vi "Return_DesiredAngle.vi"(0 "X-Position":dbl, 2 "Y-Position":dbl, 3 "Current Angle":dbl, 9 "Mining Complete":bool) -> (11 "Commence Dumping":bool, 14 "RFM":i32, 15 "RMM":i32, 16 "RRM":i32, 17 "LFM":i32, 18 "LMM":i32, 19 "LRM":i32)   [LabVIEW 2014]
panel:
  out "Desired Angle":dbl
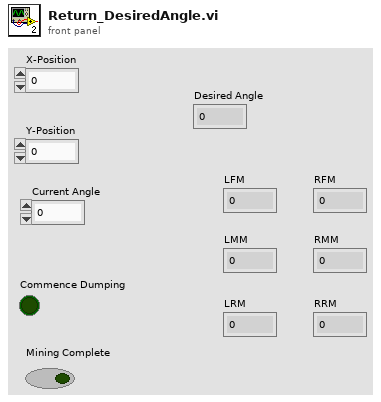
[diagram p1: front panel]
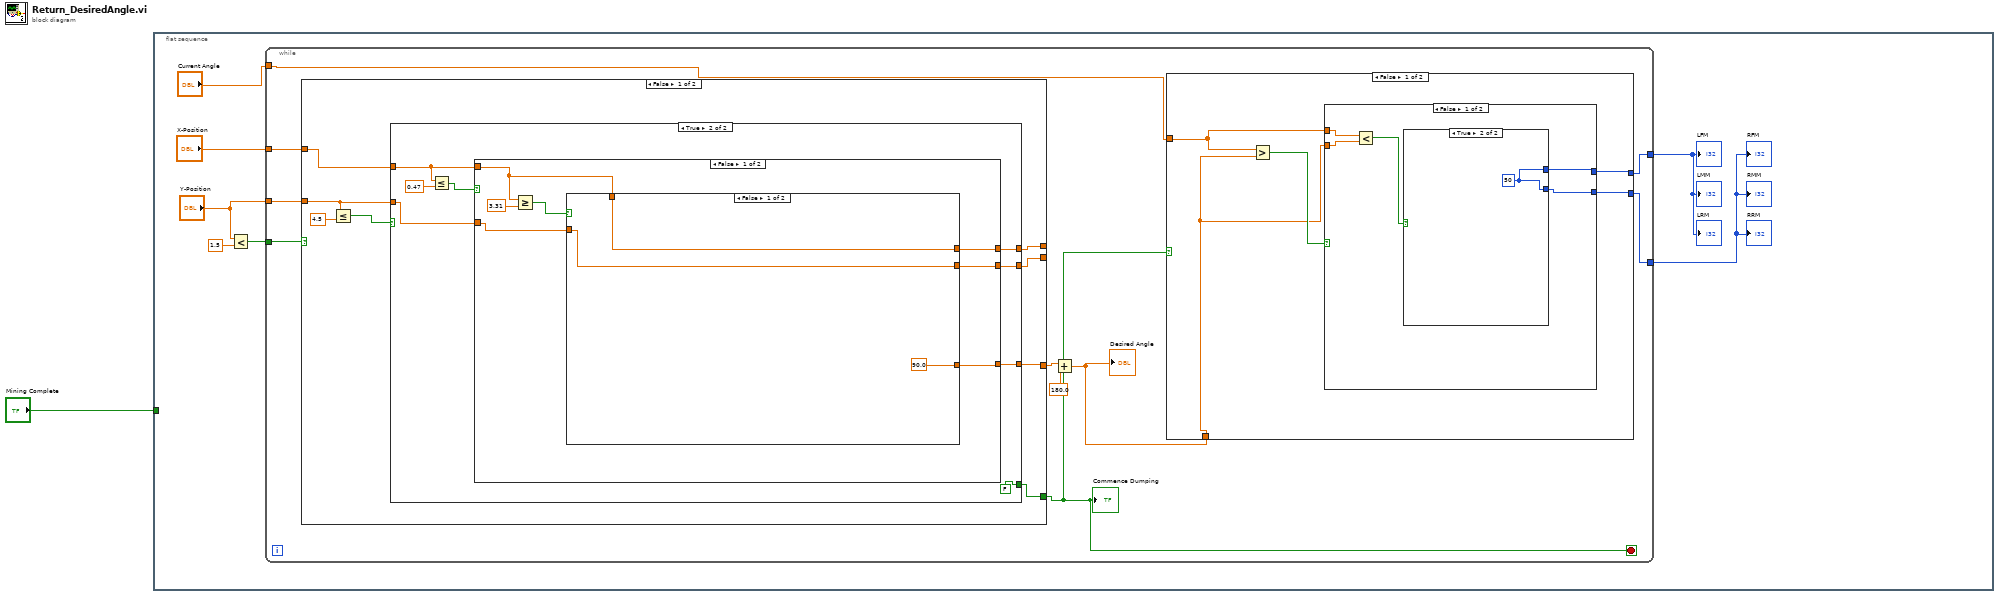
[diagram p0: block diagram]
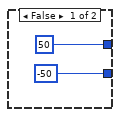
[diagram p2: hidden frame]
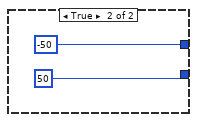
[diagram p3: hidden frame]
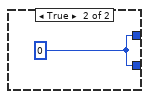
[diagram p4: hidden frame]
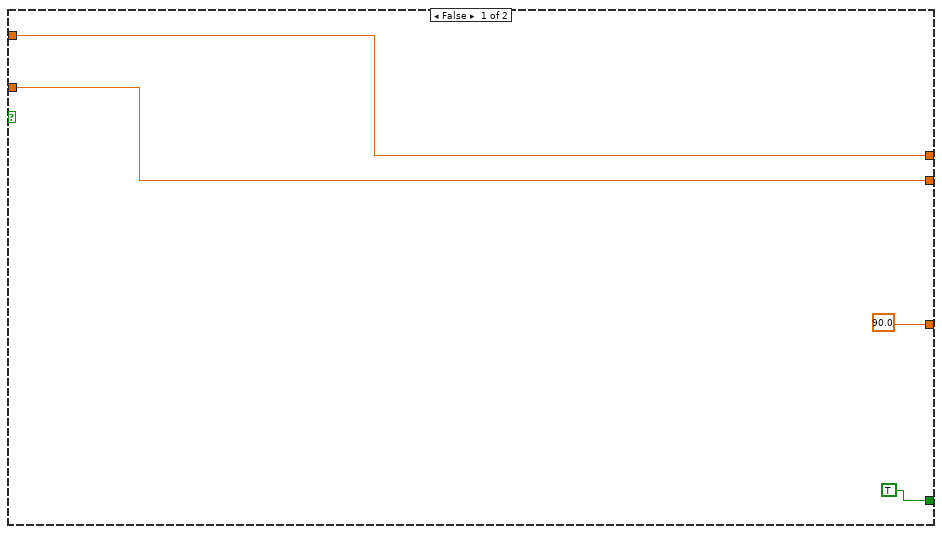
[diagram p5: hidden frame]
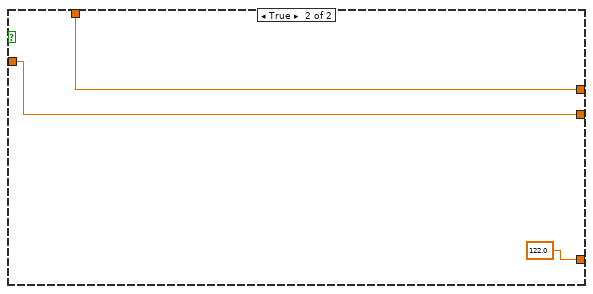
[diagram p6: hidden frame]
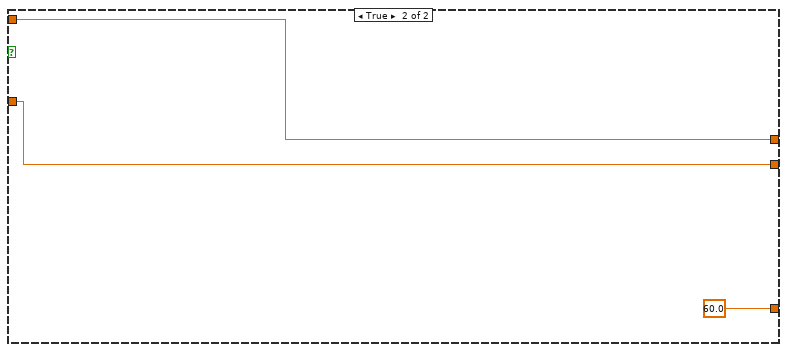
[diagram p7: hidden frame]
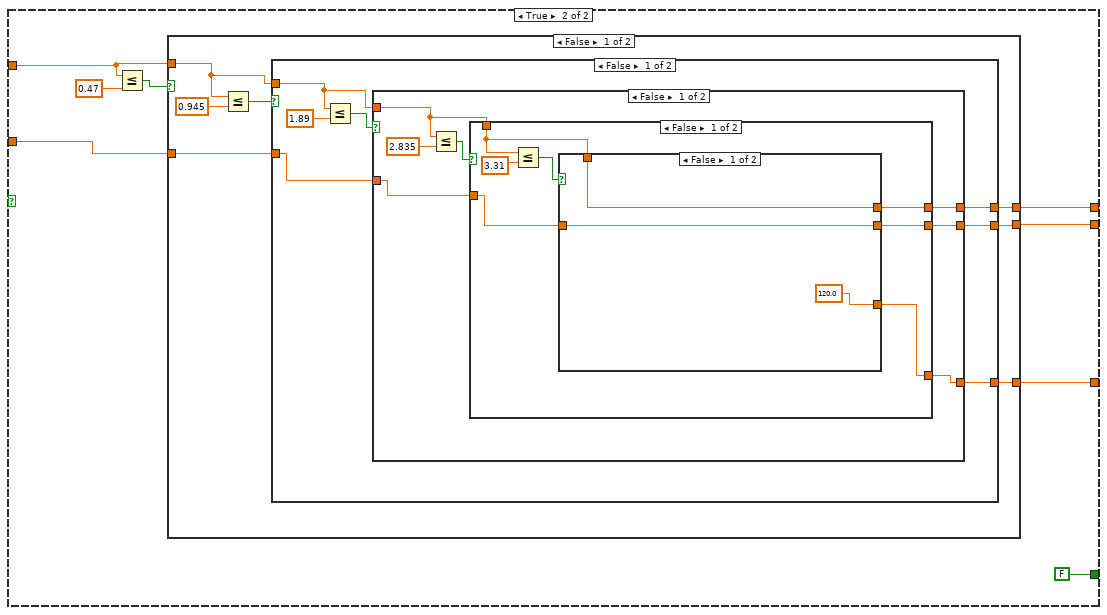
[diagram p8: hidden frame]
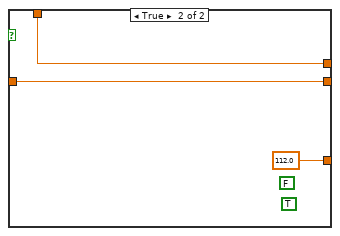
[diagram p9: hidden frame]
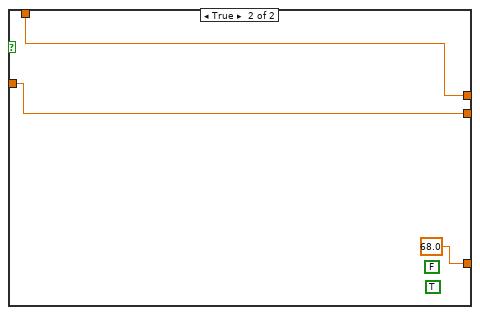
[diagram p10: hidden frame]
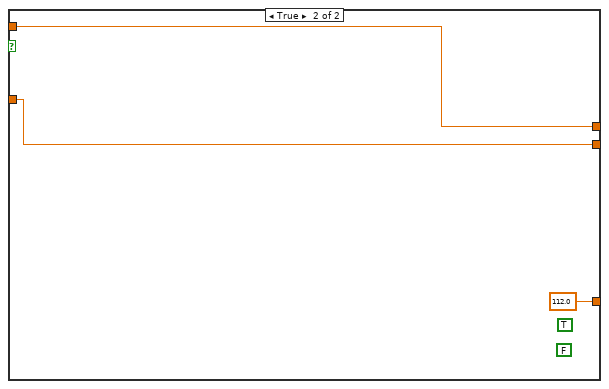
[diagram p11: hidden frame]
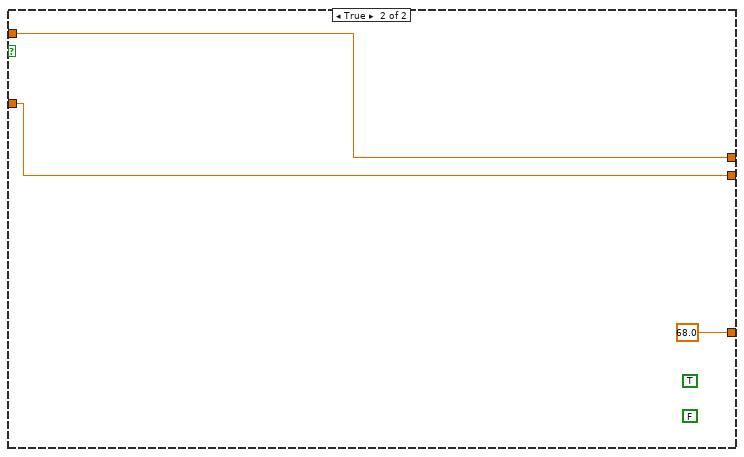
[diagram p12: hidden frame]
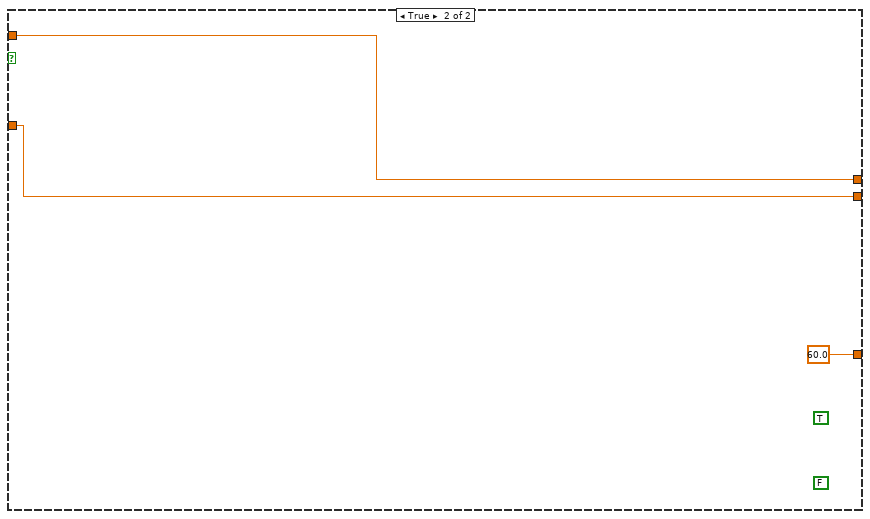
[diagram p13: hidden frame]
diagram:
  n1 = flat-sequence {
    tunnel: "Mining Complete" -> [_]
    frame #0 {
      n2 = Less?(x="Y-Position", y=1.5) -> (x < y?=w5:bool)
      n3 = while {
        tunnel: "X-Position" -> [w18]
        tunnel: "Y-Position" -> [w17]
        tunnel: w5 -> [w16]
        tunnel: "Current Angle" -> [w14]
        tunnel: [w10] -> w3
        tunnel: [w9] -> w2
        stop <- w15 stop-if-true
        n4 = case shown="False" w16 {
          tunnel: [w42 w78] -> w13
          tunnel: w18 -> [w41 w76]
          tunnel: [w36 w74] -> _
          tunnel: w17 -> [w38 w73]
          tunnel: [w37 w72] -> _
          tunnel: [w35 FALSE] -> w15
          frame False {
            n5 = Less Or Equal?(x=w38, y=4.5) -> (x <= y?=w39:bool)
            n6 = case shown="True" w39 {
              tunnel: [90.0 w52] -> w42
              tunnel: w41 -> [w45 w51]
              tunnel: w38 -> [w44 w50]
              tunnel: [w44 w49] -> w37
              tunnel: [w45 w48] -> w36
              tunnel: [TRUE FALSE] -> w35
              frame False {
              }
              frame True {
                n7 = Less Or Equal?(x=w51, y=0.47) -> (x <= y?=w53:bool)
                n8 = case shown="False" w53 {
                  tunnel: [w59 60.0] -> w52
                  tunnel: w51 -> [w58 w69]
                  tunnel: w50 -> [w57 w68]
                  tunnel: [w56 w68] -> w49
                  tunnel: [w55 w69] -> w48
                  frame False {
                    n9 = Greater Or Equal?(x=w58, y=3.31) -> (x >= y?=w60:bool)
                    n10 = case shown="False" w60 {
                      tunnel: [90.0 122.0] -> w59
                      tunnel: w58 -> [w62 w66]
                      tunnel: w57 -> [w63 w65]
                      tunnel: [w63 w65] -> w56
                      tunnel: [w62 w66] -> w55
                      frame False {
                      }
                      frame True {
                      }
                    }
                  }
                  frame True {
                  }
                }
              }
            }
          }
          frame True {
            n11 = Less Or Equal?(x=w76, y=0.47) -> (x <= y?=w75:bool)
            n12 = case shown="False" w75 {
              tunnel: w76 -> [w83 w123]
              tunnel: [w82 60.0] -> w78
              tunnel: [w81 w123] -> w74
              tunnel: w73 -> [w80 w122]
              tunnel: [w79 w122] -> w72
              frame False {
                n13 = Less Or Equal?(x=w83, y=0.945) -> (x <= y?=w85:bool)
                n14 = case shown="False" w85 {
                  tunnel: w83 -> [w90 w120]
                  tunnel: [w89 68.0] -> w82
                  tunnel: [w88 w120] -> w81
                  tunnel: w80 -> [w87 w119]
                  tunnel: [w86 w119] -> w79
                  frame False {
                    n15 = Less Or Equal?(x=w90, y=1.89) -> (x <= y?=w91:bool)
                    n16 = case shown="False" w91 {
                      tunnel: w90 -> [w97 w117]
                      tunnel: [w96 112.0] -> w89
                      tunnel: [w95 w117] -> w88
                      tunnel: w87 -> [w94 w116]
                      tunnel: [w93 w116] -> w86
                      frame False {
                        n17 = Less Or Equal?(x=w97, y=2.835) -> (x <= y?=w98:bool)
                        n18 = case shown="False" w98 {
                          tunnel: w97 -> [w104 w114]
                          tunnel: [w103 68.0] -> w96
                          tunnel: [w102 w114] -> w95
                          tunnel: w94 -> [w101 w113]
                          tunnel: [w100 w113] -> w93
                          frame False {
                            n19 = Less Or Equal?(x=w104, y=3.31) -> (x <= y?=w105:bool)
                            n20 = case shown="False" w105 {
                              tunnel: w104 -> [w108 w111]
                              tunnel: [120.0 112.0] -> w103
                              tunnel: [w108 w111] -> w102
                              tunnel: w101 -> [w107 w110]
                              tunnel: [w107 w110] -> w100
                              frame False {
                              }
                              frame True {
                                (unwired) TRUE
                                (unwired) FALSE
                              }
                            }
                          }
                          frame True {
                            (unwired) TRUE
                            (unwired) FALSE
                          }
                        }
                      }
                      frame True {
                        (unwired) FALSE
                        (unwired) TRUE
                      }
                    }
                  }
                  frame True {
                    (unwired) FALSE
                    (unwired) TRUE
                  }
                }
              }
              frame True {
                (unwired) FALSE
                (unwired) TRUE
              }
            }
          }
        }
        "Commence Dumping" <- w15
        n21 = Add(x=w13, y=180.0) -> (x+y=w12:dbl)
        "Desired Angle" <- w12
        n22 = case shown="False" w15 {
          tunnel: w14 -> [w22 _]
          tunnel: w12 -> [w21 _]
          tunnel: [w19 w34] -> w9
          tunnel: [w20 w34] -> w10
          frame False {
            n23 = Greater?(x=w22, y=w21) -> (0:w23:bool)
            n24 = case shown="False" w23 {
              tunnel: w22 -> [w28 _]
              tunnel: w21 -> [w27 _]
              tunnel: [w25 -50] -> w20
              tunnel: [w24 50] -> w19
              frame False {
                n25 = Less?(x=w28, y=w27) -> (x < y?=w26:bool)
                n26 = case shown="True" w26 {
                  tunnel: [50 w31] -> w25
                  tunnel: [-50 w31] -> w24
                  frame False {
                  }
                  frame True {
                    w31 = 50
                  }
                }
              }
              frame True {
              }
            }
          }
          frame True {
            w34 = 0
          }
        }
      }
      "LFM" <- w3
      "RFM" <- w2
      "RMM" <- w2
      "RRM" <- w2
      "LMM" <- w3
      "LRM" <- w3
    }
  }
